vi "Create UNSUBSCRIBE Packet.vi"(5 "UNSUBSCRIBE in":refnum<class "UNSUBSCRIBE.lvclass">, 8 "error in (no error)":errorcluster, 9 "Packet ID (0: generate new)":u16 format="%04x", 11 "Topic Subscriptions":string[](array[string])) -> (0 "error out":errorcluster, 3 "UNSUBSCRIBE out":refnum<class "UNSUBSCRIBE.lvclass">)   [LabVIEW 2013, in "MQTT_Control_Packets.lvlib" / "UNSUBSCRIBE.lvclass"]
uses:
  UNSUBSCRIBE.lvclass
  ControlPacket/ControlPacket.lvclass/ControlPacket.ctl
  ControlPacket/ControlPacket.lvclass
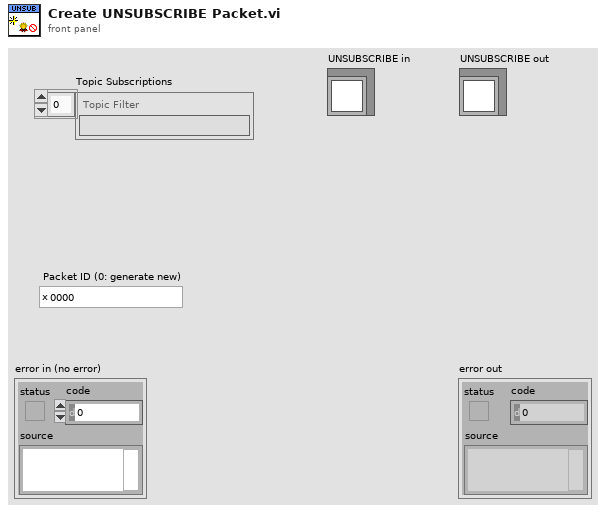
[diagram p1: front panel]
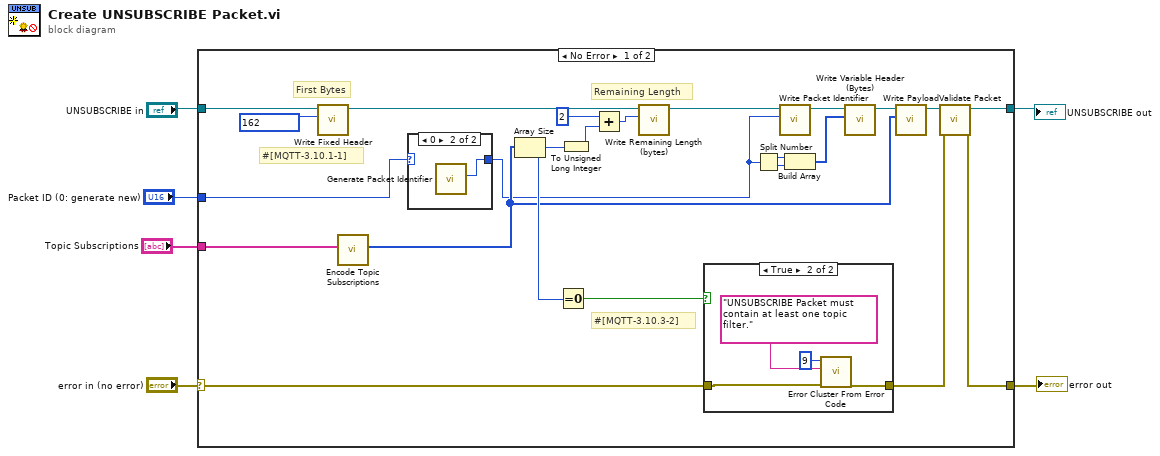
[diagram p0: block diagram]
diagram:
  n1 = case shown="No Error" "error in (no error)" {
    selector: "error in (no error)" -> [w16 w38]
    tunnel: [w11 w38] -> w2
    tunnel: [w13 w37] -> w1
    tunnel: "UNSUBSCRIBE in" -> [w29 w37]
    tunnel: "Packet ID (0: generate new)" -> [w8 _]
    tunnel: "Topic Subscriptions" -> [w10 _]
    frame No Error {
      # "#[MQTT-3.10.3-2]"
      # "#[MQTT-3.10.1-1]"
      # "Remaining Length"
      # "First Bytes"
      n2 = call "Write Fixed Header.vi"("Fixed Header"=u8 162, "ControlPacket in"=w29) -> ("ControlPacket out"=w28:refnum<class "UNSUBSCRIBE.lvclass">)  [unwired: 9 in]
      n3 = call "Encode Topic Subscriptions.vi"("Topic Subscriptions"=w10) -> ("Length-Prefixed Field"=w9:u8[])  [unwired: 10 in]
      n4 = case shown="0" w8 {
        selector: w8 -> [w30 _]
        tunnel: [w30 w31] -> w7
        frame Default {
        }
        frame 0 {
          n5 = call "Generate Packet Identifier.vi"() -> ("Packet Identifier"=w31:u16)  [unwired: 11 in]
        }
      }
      n6 = Array Size(array=w9) -> (size(s)=w17:i32)
      n7 = Equal To 0?(x=w17) -> (x = 0?=w15:bool)
      n8 = To Unsigned Long Integer(number=w17) -> (unsigned 32bit integer=w18:u32)
      n9 = Add(x=u32 2 ("Remaining Length (bytes)"), y=w18) -> (x+y=w20:u32)
      n10 = call "Write Remaining Length (bytes).vi"("Remaining Length (bytes)"=w20, "ControlPacket in"=w28) -> ("ControlPacket out"=w24:refnum<class "UNSUBSCRIBE.lvclass">)  [unwired: 9 in]
      n11 = case shown="True" w15 {
        tunnel: w16 -> [w32 w35]
        tunnel: [w32 w36] -> w12
        frame False {
        }
        frame True {
          n12 = call <vilib>:"Error Cluster From Error Code.vi"("error in (no error)"=w35, "error message (\"\")"="UNSUBSCRIBE Packet must contain at least one topic filter.", "error code (0)"=9) -> ("error out"=w36:errorcluster)  [unwired: 6 in]
        }
      }
      n13 = Split Number(x=w7) -> (hi(x)=w27:u8, lo(x)=w26:u8)
      n14 = call "Write Packet Identifier.vi"("Packet Identifier"=w7, "ControlPacket in"=w24) -> ("ControlPacket out"=w23:refnum<class "UNSUBSCRIBE.lvclass">)  [unwired: 9 in]
      n15 = Build Array(w27, w26) -> (w25:u8[])
      n16 = call "Write Variable Header (Bytes).vi"("Variable Header (Bytes)"=w25, "ControlPacket in"=w23) -> ("ControlPacket out"=w19:refnum<class "UNSUBSCRIBE.lvclass">)  [unwired: 9 in]
      n17 = call "Write Payload.vi"("Payload"=w9, "ControlPacket in"=w19) -> ("ControlPacket out"=w14:refnum<class "UNSUBSCRIBE.lvclass">)  [unwired: 9 in]
      n18 = call "Validate Packet.vi"("error in (no error)"=w12, "ControlPacket in"=w14) -> ("error out"=w11:errorcluster, "ControlPacket out"=w13:refnum<class "UNSUBSCRIBE.lvclass">)  [unwired: 8 in]
    }
    frame Error {
    }
  }
  "error out" <- w2
  "UNSUBSCRIBE out" <- w1
